vi "rad_FTP Put File Wrapper.vi"(4 "active (F)":bool, 5 "password":string, 6 "binary (T)":bool=TRUE, 7 "user (admin)":string="admin", 8 "error in (no error)":errorcluster, 9 "local path":path, 10 "remote path":string, 11 "Target settings":T1={"Hostname"="", "Serial number"="", "Product name"="", "Product code"=0, "System status"="", "Credential type"=enum."None/Unlocked", "User added?"=FALSE, "Primary NIC"={"MAC address"="", "IP Address Request Mode"=2, "IP address"="", "Subnet mask"="", "Gateway"="", "DNS server"=""}} {"Primary NIC"."IP Address Request Mode" items=["Static"=1, "DHCP/Link-Local"=2, "Link-Local Only"=4, "DHCP Only"=8]}) -> (0 "error out":errorcluster)   [LabVIEW 2023]
uses:
  Targets/TypeDefs/rad_Target Information.ctl
  Targets/TypeDefs/rad_Target Network Settings.ctl
  <vilib>/nisyscfg/Close (System).vi
  <vilib>/nisyscfg/nisyscfg.lvlib
  <vilib>/FTP/NI_FTP.lvlib
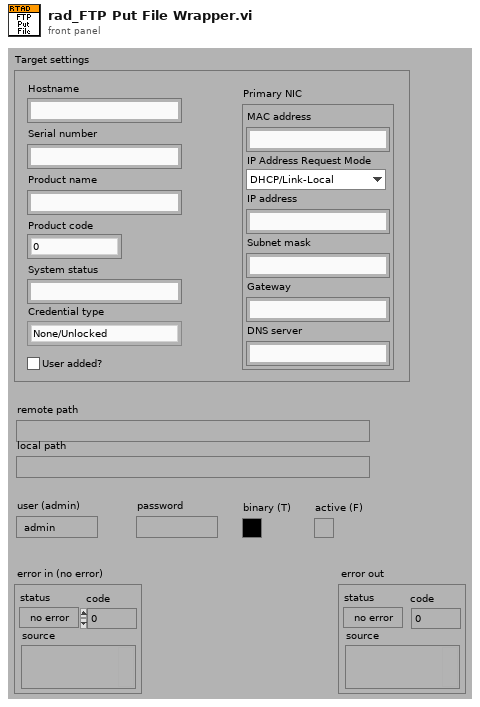
[diagram p1: front panel]
types:
  T1 = typedef "rad_Target Information.ctl" = cluster{"Hostname":string, "Serial number":string, "Product name":string, "Product code":i32, "System status":string, "Credential type":enum16{"None/Unlocked", "FTP Password", "NIAuth Credentials"}, "User added?":bool, "Primary NIC":T2}
  T2 = typedef "rad_Target Network Settings.ctl" = cluster{"MAC address":string, "IP Address Request Mode":i32, "IP address":string, "Subnet mask":string, "Gateway":string, "DNS server":string}
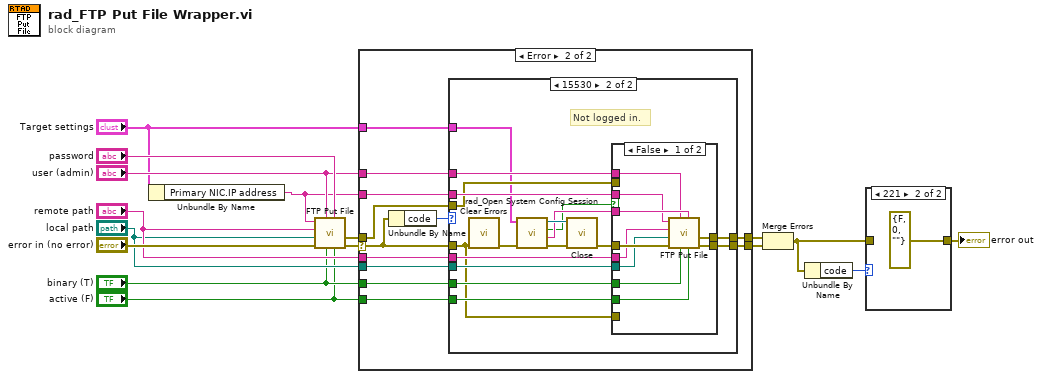
[diagram p0: block diagram]
diagram:
  n1 = Unbundle By Name("Target settings") -> ("Primary NIC.IP address"=w2:string)
  n2 = call <vilib>:"FTP Put File.vi"("active (T)"="active (F)", "password"="password", "binary (F)"="binary (T)", "user"="user (admin)", "error in (no error)"="error in (no error)", "local path"="local path", "remote path"="remote path", "host"=w2) -> ("error out"=w12:errorcluster, "file error"=w10:errorcluster)  [unwired: 2 in]
  n3 = case shown="Error" w12 {
    selector: w12 -> [w18 w24]
    tunnel: [w18 w30] -> w11
    tunnel: w2 -> [_ w29]
    tunnel: "remote path" -> [_ w28]
    tunnel: "local path" -> [_ w27]
    tunnel: "binary (T)" -> [_ w26]
    tunnel: "active (F)" -> [_ w25]
    tunnel: w10 -> [w17 w22]
    tunnel: [w17 w21] -> w4
    tunnel: "user (admin)" -> [_ w20]
    tunnel: "Target settings" -> [_ w19]
    frame No Error {
    }
    frame Error {
      n4 = Unbundle By Name(w24) -> ("code"=w23:i32)
      n5 = case shown="15530" w23 {
        tunnel: w24 -> [w32 w37]
        tunnel: [w32 w45] -> w30
        tunnel: w29 -> [_ w43]
        tunnel: w28 -> [_ w42]
        tunnel: w27 -> [_ w41]
        tunnel: w26 -> [_ w40]
        tunnel: w25 -> [_ w39]
        tunnel: w22 -> [w31 w36]
        tunnel: [w31 w35] -> w21
        tunnel: w20 -> [_ w34]
        tunnel: w19 -> [_ w33]
        frame Default {
        }
        frame 15530 {
          # "Not logged in."
          n6 = call <vilib>:"Clear Errors.vi"("error in (no error)"=w37) -> ("error out"=w47:errorcluster)  [unwired: 5 in, 1 out]
          n7 = call "rad_Open System Config Session.vi"("error in (no error)"=w47, "Target settings"=w33) -> ("error out"=w48:errorcluster, "Password out"=w44:string, "Cancelled"=w38:bool, "Session out"=w49:refnum<k21>)  [unwired: 6 in]
          n8 = call-poly <vilib>:"Close.vi"("error in (no error)"=w48, "Session in"=w49) -> ("error out"=w46:errorcluster)  [unwired: 9 in]
          n9 = case shown="False" w38 {
            tunnel: w46 -> [w58 _]
            tunnel: [w59 w61] -> w45
            tunnel: w44 -> [w56 _]
            tunnel: w43 -> [w54 _]
            tunnel: w42 -> [w55 _]
            tunnel: w41 -> [w53 _]
            tunnel: w40 -> [w52 _]
            tunnel: w39 -> [w51 _]
            tunnel: w37 -> [_ w61]
            tunnel: [w57 w60] -> w35
            tunnel: w36 -> [_ w60]
            tunnel: w34 -> [w50 _]
            frame False {
              n10 = call <vilib>:"FTP Put File.vi"("active (T)"=w51, "password"=w56, "binary (F)"=w52, "user"=w50, "error in (no error)"=w58, "local path"=w53, "remote path"=w55, "host"=w54) -> ("error out"=w59:errorcluster, "file error"=w57:errorcluster)  [unwired: 2 in]
            }
            frame True {
            }
          }
        }
      }
    }
  }
  n11 = Merge Errors(w4, w11) -> (w13:errorcluster)
  n12 = Unbundle By Name(w13) -> ("code"=w14:i32)
  n13 = case shown="221" w14 {
    tunnel: w13 -> [w62 _]
    tunnel: [w62 errorcluster {"status"=FALSE, "code"=0, "source"=""} ("error IO")] -> w15
    frame Default {
    }
    frame 221 {
    }
  }
  "error out" <- w15
